vi "mlink_error.vi"(8 "error in (no error)":errorcluster, 11 "error code":i32) -> (0 "error out":errorcluster)   [LabVIEW 2009, in "MicroDAQ.lvlib" / "mlink.lvlib"]
doc: "This function returns error description for the given MLink error code."
uses:
  <instrlib>/MicroDAQ/Mlink library wraper/mlink.lvlib
  <instrlib>/MicroDAQ/MLink32.dll
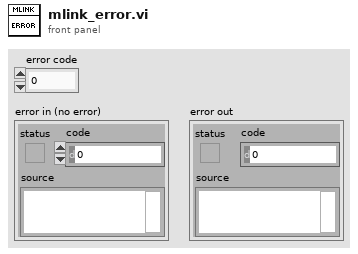
[diagram p1: front panel]
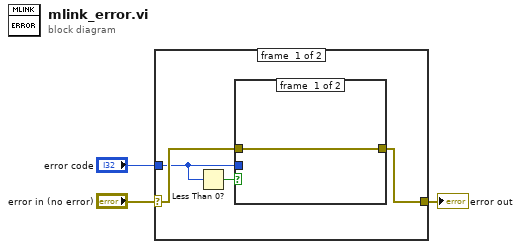
[diagram p0: block diagram]
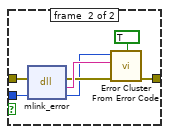
[diagram p2: hidden frame]
diagram:
  n1 = case shown="No Error" "error in (no error)" {
    selector: "error in (no error)" -> [w6 w16]
    tunnel: [w4 w16] -> w3
    tunnel: "error code" -> [w5 _]
    frame #0 {
      n2 = Less Than 0?(x=w5) -> (x < 0?=w7:bool)
      n3 = case shown="True" w7 {
        tunnel: w6 -> [w8 w12]
        tunnel: w5 -> [_ w10]
        tunnel: [w8 w15] -> w4
        frame #0 {
        }
        frame #1 {
          n4 = dll-call lib="C:/Program Files (x86)/National Instruments/LabVIEW 2009/instr.lib/MicroDAQ/MLink32.dll" fn="mlink_error"(error in=w12, "Error number"=w10) -> (error out=w11:errorcluster, "return type"=w13:string, "Error number"=w9:i32)  [unwired: 2 in, 1 out]
          n5 = call <vilib>:"Error Cluster From Error Code.vi"("show call chain? (False)"=TRUE, "error in (no error)"=w11, "error message (\"\")"=w13, "error code (0)"=w9) -> ("error out"=w15:errorcluster)  [unwired: 5 in]
        }
      }
    }
    frame #1 {
    }
  }
  "error out" <- w3
